vi "NIDCPower_channel_ganging - fetch multiple.vi"(0 "Ganged Session In":T1, 7 "Count":i32, 9 "timeout (1.0)":dbl=1.0 format="%.6p", 11 "error in (no error)":errorcluster) -> (2 "Ganged Voltage Measurement":dbl[](array[numeric]), 3 "Ganged Current Measurement":dbl[](array[numeric]), 4 "Ganged Session Out":T1, 6 "voltage measurements":dbl[][](array[numeric]) format="%#_6p", 8 "current measurements":dbl[][](array[numeric]) format="%#_6p", 10 "in compliance":bool[][](array[boolean]), 14 "Measure Record dt":dbl[](array[numeric]), 15 "error out":errorcluster)   [LabVIEW 2021]
uses:
  ctl/NIDCPower_channel_ganging - ctl - ganged session.ctl
  ctl/NIDCPower_channel_ganging - ctl - ganged config.ctl
  ctl/NIDCPower_channel_ganging - ctl - channel mode.ctl
panel:
  out "Waveform Graph":dbl[](graph)
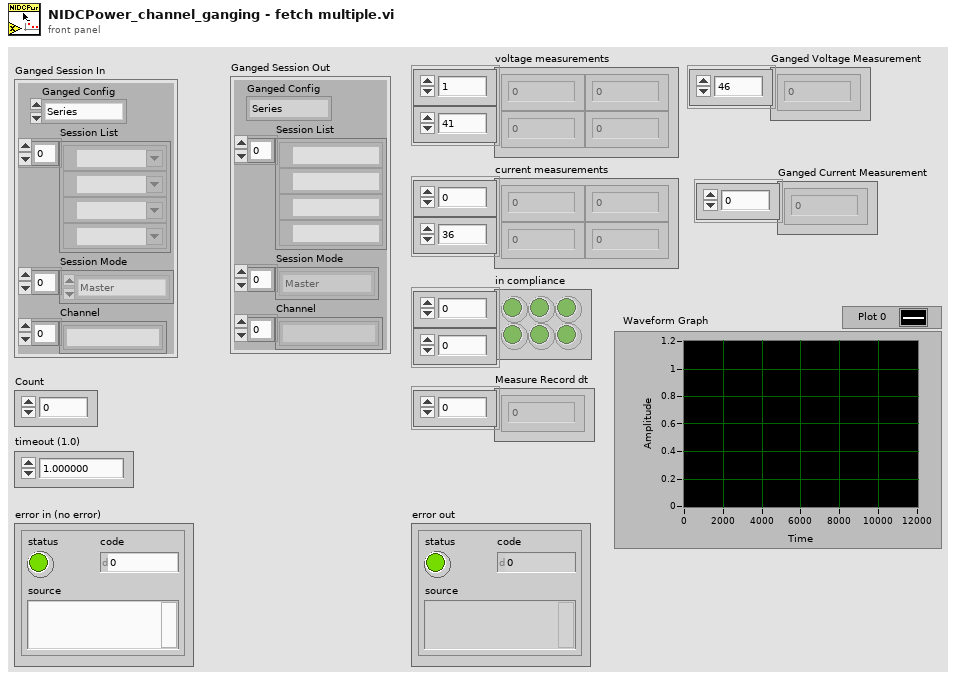
[diagram p1: front panel]
types:
  T1 = typedef "NIDCPower_channel_ganging - ctl - ganged session.ctl" = cluster{"Ganged Config":T2, "Session List":refnum<k15>[], "Session Mode":T3[], "Channel":string[]}
  T2 = typedef "NIDCPower_channel_ganging - ctl - ganged config.ctl" = enum32{"Series", "Parallel", "Manual"}
  T3 = typedef "NIDCPower_channel_ganging - ctl - channel mode.ctl" = enum32{"Master", "Slave", "Slave - Inverted"}
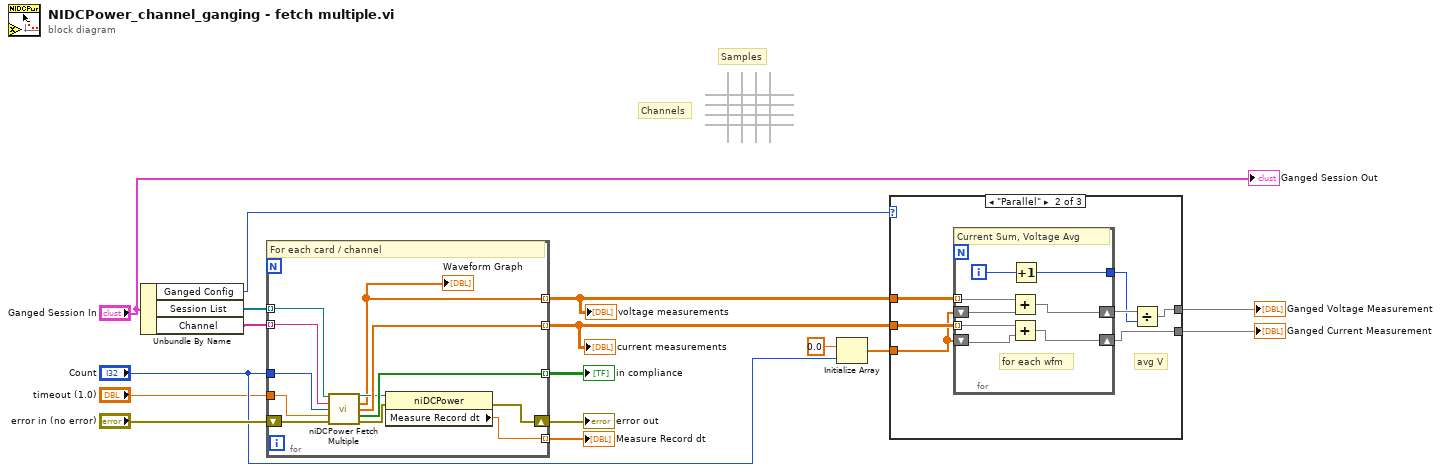
[diagram p0: block diagram]
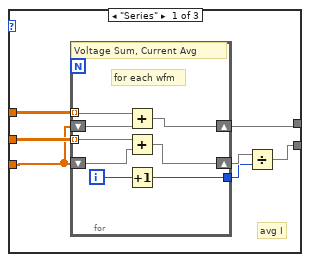
[diagram p2: hidden frame]
diagram:
  # "Channels"
  # "Samples"
  n1 = Unbundle By Name("Ganged Session In") -> ("Ganged Config"=w1:T2, "Session List"=w13:refnum<k15>[], "Channel"=w15:string[])
  n2 = for {
    tunnel: w13 -> [w27] mode=indexing
    shift-right: [w23] -> w12
    shift-left: "error in (no error)" -> [w26]
    tunnel: "Count" -> [w28]
    tunnel: w15 -> [w18] mode=indexing
    tunnel: [w19] -> w3 mode=indexing
    tunnel: [w25] -> w6 mode=indexing
    tunnel: [w24] -> w11 mode=indexing
    tunnel: [w20] -> w10 mode=indexing
    tunnel: "timeout (1.0)" -> [w17]
    # "For each card / channel"
    n3 = call <instrlib>:"niDCPower Fetch Multiple.vi"("instrument handle"=w27, "channel name"=w18, "count (1)"=w28, "timeout (1.0)"=w17, "error in (no error)"=w26) -> ("instrument handle out"=w22:refnum<k15>, "voltage measurements"=w19:dbl[], "current measurements"=w25:dbl[], "in compliance"=w24:bool[], "error out"=w21:errorcluster)  [unwired: 5 in, 1 out]
    "Waveform Graph" <- w19
    n4 = property class="niDCPower"(reference=w22, error in=w21) -> (error out=w23:errorcluster, "Measure Record dt"=w20:dbl)  [unwired: 1 out]
  }
  "error out" <- w12
  "in compliance" <- w11
  "current measurements" <- w6
  "voltage measurements" <- w3
  "Measure Record dt" <- w10
  n5 = Initialize Array(0.0 ("element"), "Count") -> (w7:dbl[])
  n6 = case shown="\"Parallel\"" w1 {
    tunnel: w6 -> [w34 w50 _]
    tunnel: [w29 w49 _] -> w5
    tunnel: [w32 w44 _] -> w4
    tunnel: w3 -> [w35 w48 _]
    tunnel: w7 -> [w33 w47 _]
    frame "Series" {
      # "avg I"
      n7 = for {
        shift-right: [w41] -> w31
        shift-left: w33 -> [w43]
        tunnel: w34 -> [w42] mode=indexing
        tunnel: w35 -> [w40] mode=indexing
        shift-right: [w38] -> w32
        shift-left: w33 -> [w39]
        tunnel: [w36] -> w30
        i -> [w37]
        # "for each wfm"
        # "Voltage Sum, Current Avg"
        n8 = Add(x=w40, y=w39) -> (x+y=w38:dbl[])
        n9 = Add(x=w42, y=w43) -> (x+y=w41:dbl[])
        n10 = Increment(x=w37) -> (x+1=w36:i32)
      }
      n11 = Divide(x=w31, y=w30) -> (x/y=w29:dbl[])
    }
    frame "Parallel" {
      # "avg V"
      n12 = for {
        shift-right: [w56] -> w49
        shift-left: w47 -> [w58]
        tunnel: w50 -> [w57] mode=indexing
        tunnel: w48 -> [w55] mode=indexing
        shift-right: [w53] -> w46
        shift-left: w47 -> [w54]
        tunnel: [w51] -> w45
        i -> [w52]
        # "for each wfm"
        # "Current Sum, Voltage Avg"
        n13 = Add(x=w55, y=w54) -> (x+y=w53:dbl[])
        n14 = Add(x=w57, y=w58) -> (x+y=w56:dbl[])
        n15 = Increment(x=w52) -> (x+1=w51:i32)
      }
      n16 = Divide(x=w46, y=w45) -> (x/y=w44:dbl[])
    }
    frame "Manual" {
    }
  }
  "Ganged Current Measurement" <- w5
  "Ganged Voltage Measurement" <- w4
  "Ganged Session Out" <- "Ganged Session In"
